vi "3.0-FPGA Functional Global.vi"(2 "Ref In":T1, 3 "Enum":enum16{"Start", "End", "Borrow", "Return"}(ring)) -> (0 "Ref Out":T1, 1 "Has Refrence":bool)   [LabVIEW 2010]
uses:
  2-Low Neurons/2-FPGA VI Typedef.ctl
  2-Low Neurons/2.1-Act Command Typedef.ctl
  2-Low Neurons/2.1 PID Gains Typedef.ctl
  <vilib>/userDefined/High Color/nirio_resource_hc.ctl
  <vilib>/rvi/interface/nirviOpenFPGA/nirviOpenFPGA.xnode
  FPGA Bitfiles/DaveBrain_FPGATarget_1-Hindbrain_F0E489D8.lvbitx
  1-Hindbrain.vi
  <vilib>/rvi/ClientSDK/nirviWhatTheDeviceIsDoing.ctl
  <vilib>/rvi/interface/nirviReadWriteControl/nirviReadWriteControl.xnode
  <vilib>/rvi/interface/common/niFpgaNodeNameForErrorReporting.ctl
  <vilib>/rvi/errors/niLvFpgaWhatHappensToTopLevelVI.ctl
  <vilib>/rvi/interface/nirviCloseFPGA/nirviCloseFPGA.xnode
  <vilib>/FPGAPlugInAG/cRIO-9104/niLvFpga_Open_cRIO-9104.vi
  <vilib>/Utility/error.llb/Error Cluster From Error Code.vi
  <vilib>/rvi/errors/niLvFpgaAdjustHostInterfaceError.vi
  <vilib>/FPGAPlugInAG/cRIO-9104/niLvFpga_Close_cRIO-9104.vi
  NiFpgaLv.dll
panel:
  out "error out 2":errorcluster
  out "error out":errorcluster
  out "Pointer to FPGA":u32
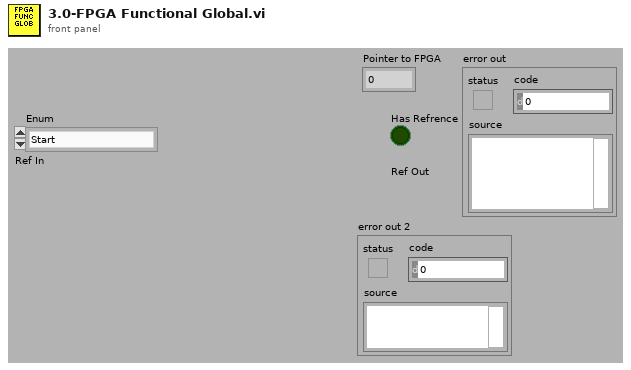
[diagram p1: front panel]
types:
  T1 = typedef "2-FPGA VI Typedef.ctl" = refnum<k20>
  T2 = typedef "2.1-Act Command Typedef.ctl" = cluster{"Inhibit All Motors":bool, "2.1 Direct Override":bool, "Drive Speed Integer Setpoint":i32, "Steering Integer Setpoint":i32, "Lidar Position Integer Setpoint":i32, "Drive Direct":fxp<+/-,20,5>, "Steer Direct":fxp<+/-,20,5>, "Lidar Direct ":fxp<+/-,20,5>, "2.1.3 Drive PID Gains":T3, "2.1.3 Steering PID Gains":T3, "Drive Limit":fxp<+/-,20,5>, "2.1.3 Steering V PID":T3, "Steering V Magnitude":i16}
  T3 = typedef "2.1 PID Gains Typedef.ctl" = cluster{"P Gain":fxp<+/-,18,1>, "I Gain":fxp<+/-,18,1>, "D Gain":fxp<+/-,18,1>, "P Gain - Exp":i8, "I Gain - Exp":i8, "D Gain - Exp":i8, "I Saturate":fxp<+/-,64,46>}
  T4 = typedef "niFpgaNodeNameForErrorReporting.ctl" = enum16{"Open FPGA VI Reference", "Read/Write Control", "Invoke Method: Abort", "Invoke Method: Acknowledge IRQ", "Invoke Method: Download", "Invoke Method: FIFO.Configure", "Invoke Method: FIFO.Read", "Invoke Method: FIFO.Start", "Invoke Method: FIFO.Stop", "Invoke Method: FIFO.Write", "Invoke Method: Reset", "Invoke Method: Run", "Invoke Method: Wait on IRQ", "Close FPGA VI Reference"}
  T5 = typedef "niLvFpgaWhatHappensToTopLevelVI.ctl" = enum16{"top level VI scripted behind XNode", "top level VI inlined behind XNode"}
  T6 = typedef "nirviWhatTheDeviceIsDoing.ctl" = enum32{"nothing", "something other than LabVIEW FPGA", "FPGA interface", "interactive", "emulation"}
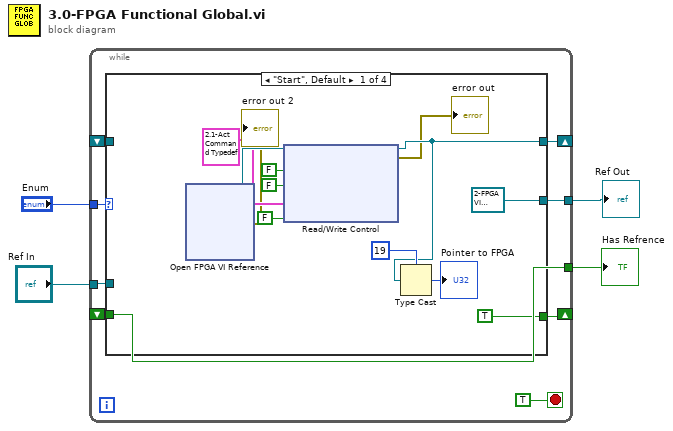
[diagram p0: block diagram]
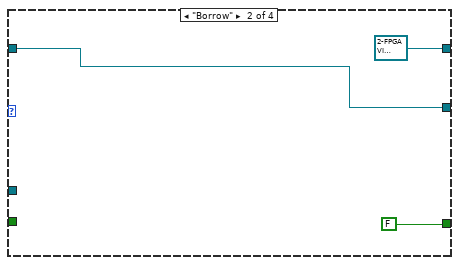
[diagram p2: hidden frame]
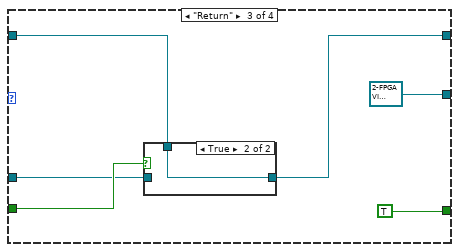
[diagram p3: hidden frame]
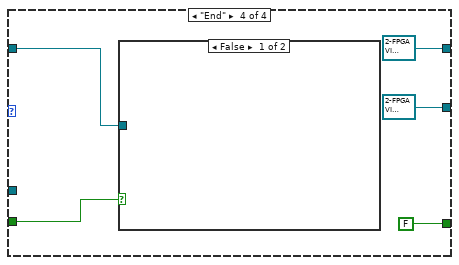
[diagram p5: hidden frame]
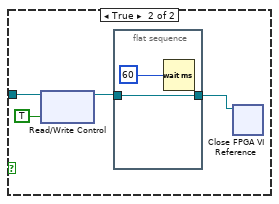
[diagram p6: hidden frame]
diagram:
  n1 = while {
    shift-right: [w9] -> _
    shift-left: _ -> [w8]
    tunnel: "Enum" -> [w11]
    tunnel: "Ref In" -> [w10]
    shift-right: [w7] -> _
    shift-left: _ -> [w5]
    tunnel: [w6] -> w2
    tunnel: [w5] -> w1
    stop <- TRUE stop-if-true
    n2 = case shown="\"Start\", Default" w11 {
      tunnel: w10 -> [_ _ w149 _]
      tunnel: [w16 T1 refnum ("Ref In") w150 T1 refnum ("Ref In")] -> w9
      tunnel: w8 -> [_ w146 w148 w159]
      tunnel: [TRUE FALSE TRUE FALSE] -> w7
      tunnel: w5 -> [_ _ w151 w158]
      tunnel: [T1 refnum ("Ref In") w146 T1 refnum ("Ref In") T1 refnum ("Ref In")] -> w6
      frame "Start", Default {
        n3 = xnode "Open FPGA VI Reference"() -> ("FPGA VI Reference Out"=w23:T1, "error out"=→"error out 2":errorcluster)  [unwired: 2 in]
        n4 = xnode "Read/Write Control"("FPGA VI Reference In"=w23, "Begin"=FALSE, "Restart"=FALSE, "2.1 Act Command"=T2 {"Inhibit All Motors"=TRUE, "2.1 Direct Override"=TRUE, "Drive Speed Integer Setpoint"=0, "Steering Integer Setpoint"=0, "Lidar Position Integer Setpoint"=0, "Drive Direct"=0.0, "Steer Direct"=0.0, "Lidar Direct "=0.0, "2.1.3 Drive PID Gains"={"P Gain"=0.25, "I Gain"=0.25, "D Gain"=0.25, "P Gain - Exp"=2, "I Gain - Exp"=2, "D Gain - Exp"=2, "I Saturate"=0.25}, "2.1.3 Steering PID Gains"={"P Gain"=-0.34999847412109375, "I Gain"=-0.5999984741210938, "D Gain"=-0.5, "P Gain - Exp"=5, "I Gain - Exp"=4, "D Gain - Exp"=11, "I Saturate"=0.02500152587890625}, "Drive Limit"=0.0, "2.1.3 Steering V PID"={"P Gain"=0.0, "I Gain"=0.0, "D Gain"=0.0, "P Gain - Exp"=0, "I Gain - Exp"=0, "D Gain - Exp"=0, "I Saturate"=0.0}, "Steering V Magnitude"=0}, "stop"=FALSE) -> ("FPGA VI Reference Out"=w16:T1, "error out"=→"error out":errorcluster)  [unwired: 1 in]
        n5 = Type Cast(type=u32 19 ("millisecond multiple"), x=w16) -> (*(type *) &x=→"Pointer to FPGA":u32)
      }
      frame "Borrow" {
      }
      frame "Return" {
        n6 = case shown="True" w151 {
          tunnel: [w153 w154] -> w150
          tunnel: w149 -> [w153 _]
          tunnel: w148 -> [_ w154]
          frame False {
          }
          frame True {
          }
        }
      }
      frame "End" {
        n7 = case shown="False" w158 {
          tunnel: w159 -> [_ w162]
          frame False {
          }
          frame True {
            n8 = xnode "Read/Write Control"("FPGA VI Reference In"=w162, "stop"=TRUE) -> ("FPGA VI Reference Out"=w160:T1)  [unwired: 1 in, 1 out]
            n9 = flat-sequence {
              tunnel: [w164] -> w161
              tunnel: w160 -> [w164]
              frame #0 {
                n10 = Wait (ms)(milliseconds to wait=u32 60) -> ()  [unwired: 1 out]
              }
            }
            n11 = xnode "Close FPGA VI Reference"("FPGA VI Reference In"=w161) -> ()  [unwired: 1 in, 1 out]
          }
        }
      }
    }
  }
  "Ref Out" <- w2
  "Has Refrence" <- w1
